vi "Write Bandwidth (nm).vi"(8 "error in (no error)":errorcluster, 10 "Bandwidth (nm)":dbl, 11 "Spectrometer in":refnum<class "Spectrometer.lvclass">) -> (0 "error out":errorcluster, 3 "Spectrometer out":refnum<class "Spectrometer.lvclass">)   [LabVIEW 2017, in "Spectrometer.lvclass"]
uses:
  Spectrometer.lvclass
  Spectrometer.lvclass/Spectrometer.ctl
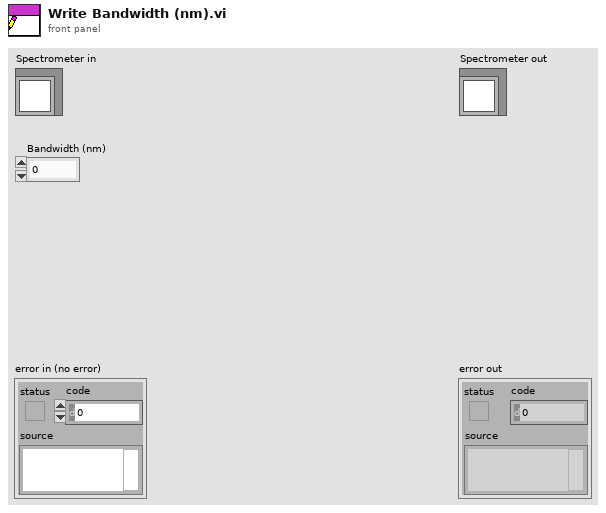
[diagram p1: front panel]
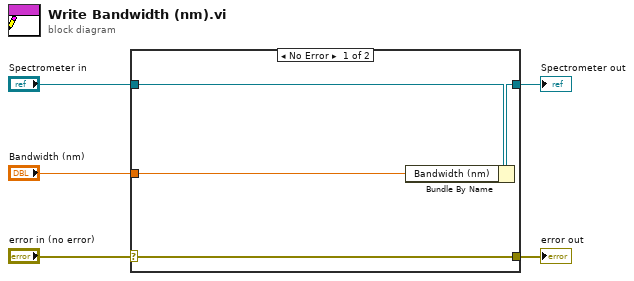
[diagram p0: block diagram]
diagram:
  n1 = case shown="No Error" "error in (no error)" {
    selector: "error in (no error)" -> [w9 w10]
    tunnel: [w9 w10] -> w4
    tunnel: [w7 w11] -> w2
    tunnel: "Spectrometer in" -> [w8 w11]
    tunnel: "Bandwidth (nm)" -> [w6 _]
    frame No Error {
      n2 = Bundle By Name(cluster=w8, "Bandwidth (nm)"=w6) -> (w7:refnum<class "Spectrometer.lvclass">)
    }
    frame Error {
    }
  }
  "error out" <- w4
  "Spectrometer out" <- w2
